vi "Initialize.vi"(8 "Error In":errorcluster, 11 "VISA name":refnum<visa-resource-name>) -> (0 "Error Out":errorcluster)   [LabVIEW 2019, in "IDEX.lvlib"]
uses:
  IDEX.lvlib
  Queues/Queues.lvlib
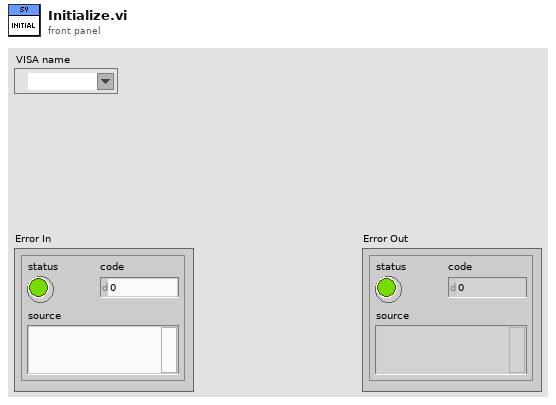
[diagram p1: front panel]
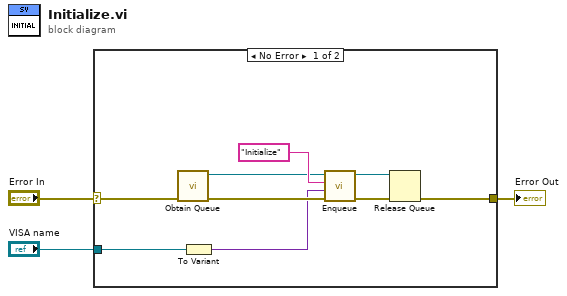
[diagram p0: block diagram]
diagram:
  n1 = case shown="No Error" "Error In" {
    selector: "Error In" -> [w11 w13]
    tunnel: [w5 w13] -> w3
    tunnel: "VISA name" -> [w8 _]
    frame No Error {
      n2 = call "Obtain Queue.vi"("Error In"=w11) -> ("Error Out"=w10:errorcluster, "Queue out"=w9:refnum<queue>)  [unwired: 9 in]
      n3 = To Variant(anything=w8) -> (Variant=w7:variant)
      n4 = call "Enqueue.vi"("Error In"=w10, "Data"=w7, "State"="Initialize", "Queue in"=w9) -> ("Error Out"=w6:errorcluster, "Queue out"=w4:refnum<queue>)  [unwired: 6 in]
      n5 = Release Queue(queue=w4, error in (no error)=w6) -> (error out=w5:errorcluster)  [unwired: 1 in, 2 out]
    }
    frame Error {
    }
  }
  "Error Out" <- w3
